vi "_Raise Source Changed Event.vi"(4 "WebView2.lvlib:WebView2 Control.lvclass":refnum<class "WebView2 Control.lvclass">, 5 "Event Data":cluster{"sender":refnum<k24>, "e":refnum<k24>}, 6 "Control Ref":refnum<k24>, 7 "Event Common Data":T1) -> ()   [LabVIEW 2020, in "WebView2.lvlib" / "WebView2 Control.lvclass"]
uses:
  WebView2 Control.lvclass
  C:/Users/Simon/Documents/GitHub/LV-WebView2/Source/Libs/Microsoft.Web.WebView2.Core.dll
  Libs/Microsoft.Web.WebView2.Core.dll
  Source Changed Event Data.ctl
  WebView2 Control.lvclass/WebView2 Control.ctl
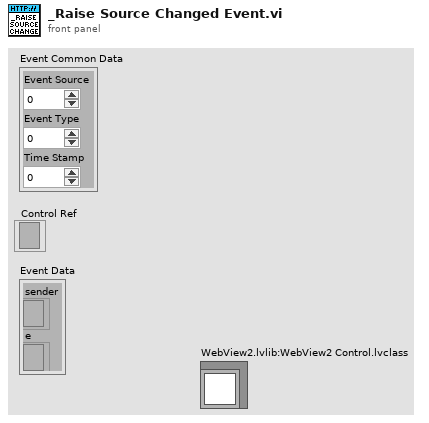
[diagram p1: front panel]
types:
  T1 = cluster{"Event Source":i32, "Event Type":u32, "Time Stamp":u32}
  T2 = typedef "WebView2.lvlib/WebView2 Control.lvclass/Source Changed Event Data.ctl" = cluster{"Source":string, "IsNewDocument":bool}
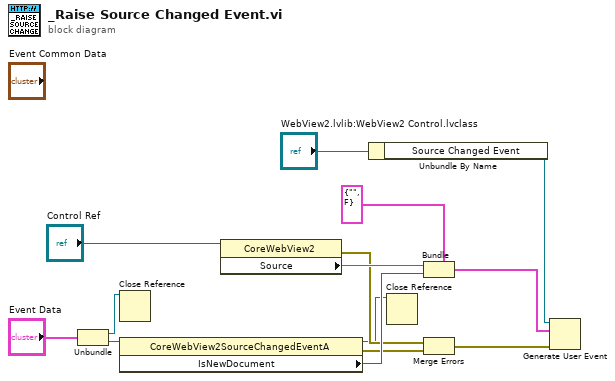
[diagram p0: block diagram]
diagram:
  n1 = Unbundle("Event Data") -> ("sender"=w2:refnum<k24>, "e"=w11:refnum<k24>)
  n2 = Close Reference(reference=w2) -> ()  [unwired: 1 in, 1 out]
  n3 = property class="CoreWebView2SourceChangedEventA"(reference=w11) -> (reference out=w1:refnum<k24>, error out=w5:errorcluster, "IsNewDocument"=w9:bool)  [unwired: 1 in]
  n4 = property class="CoreWebView2"(reference="Control Ref") -> (error out=w3:errorcluster, "Source"=w7:string)  [unwired: 1 in, 1 out]
  n5 = Unbundle By Name("WebView2.lvlib:WebView2 Control.lvclass") -> ("Source Changed Event"=w13:refnum<user-event>)
  n6 = Close Reference(reference=w1) -> ()  [unwired: 1 in, 1 out]
  n7 = Bundle(cluster=T2 {"Source"="", "IsNewDocument"=FALSE} ("output cluster"), "Source"=w7, "IsNewDocument"=w9) -> (w6:T2)
  n8 = Merge Errors(w3, w5) -> (w4:errorcluster)
  n9 = Generate User Event(user event=w13, event data cluster=w6, error in=w4) -> ()  [unwired: 1 in, 2 out]
